vi "slope corrector.vi"(8 "Pump Calibration":T1, 11 "flow rate":dbl[unit]) -> (3 "modified flow rate":dbl[unit])   [LabVIEW 2012]
uses:
  calibration values.ctl
  <vilib>/Analysis/NI_AALPro.lvlib
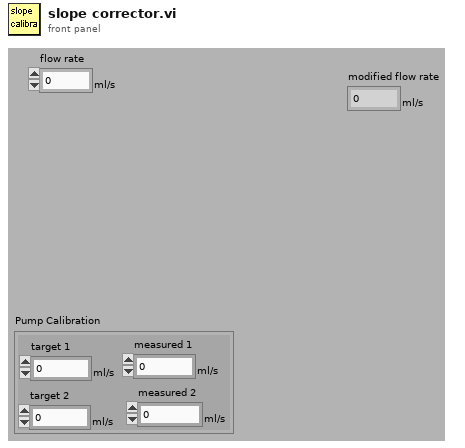
[diagram p1: front panel]
types:
  T1 = typedef "calibration values.ctl" = cluster{"target 1":dbl[unit], "target 2":dbl[unit], "measured 1":dbl[unit], "measured 2":dbl[unit]}
  T2 = cluster{"target 1":dbl, "target 2":dbl, "measured 1":dbl, "measured 2":dbl}
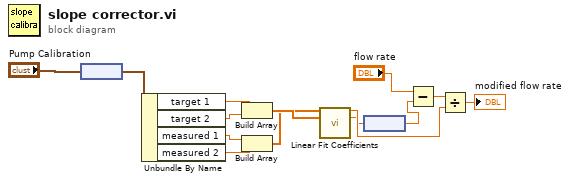
[diagram p0: block diagram]
diagram:
  n1 = node("Pump Calibration") -> (w7:T2)
  n2 = Unbundle By Name(w7) -> ("target 1"=w13:dbl, "target 2"=w12:dbl, "measured 1"=w11:dbl, "measured 2"=w10:dbl)
  n3 = Build Array(w13, w12) -> (w9:dbl[])
  n4 = Build Array(w11, w10) -> (w8:dbl[])
  n5 = call <vilib>:"Linear Fit Coefficients.vi"("Y"=w8, "X"=w9) -> ("slope"=w2:dbl, "intercept"=w1:dbl)  [unwired: 11 in, 1 out]
  n6 = node(w1) -> (w5:dbl[unit])
  n7 = Subtract(x="flow rate", y=w5) -> (x-y=w4:dbl[unit])
  n8 = Divide(x=w4, y=w2) -> (x/y=→"modified flow rate":dbl[unit])
